vi "Refnum Names.vi"() -> ()   [LabVIEW 2015]
panel:
  in  "Arm":string
  in  "Indexer":string="Gyro"
  in  "Piston":string="Mast"
  in  "Shooter":string="Arm"
  in  "Drive Motors":string="Drive"
  in  "Joystick W/Rotation":string="Joystick 0"
  # "Motors"
  # "Solenoids"
  # "Joysticks"
  # "Relays"
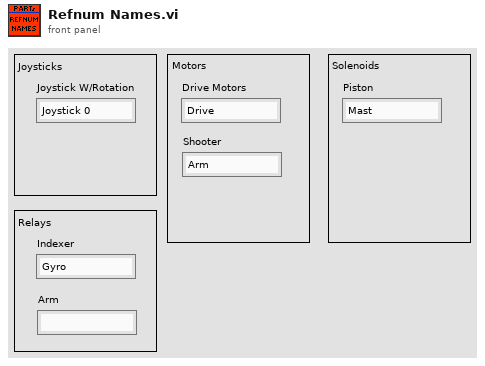
[diagram p1: front panel]
diagram:
